vi "xdevice.vi"() -> ()   [LabVIEW 2019]
panel:
  out "GetDeviceInterface":refnum<k7>
  in  "stop":bool
  out "Device moved":bool
  in  "Wavelength":dbl=795.0
  out "Temperature":dbl
  out "Serial number":string
  out "Wavelength":dbl
  out "Angle":dbl
  out "Device detected":bool
  out "Error message":string
  in  "xphyspecLib.IXPhySpec":refnum<k7>
  # "Device status"
  # "Device information"
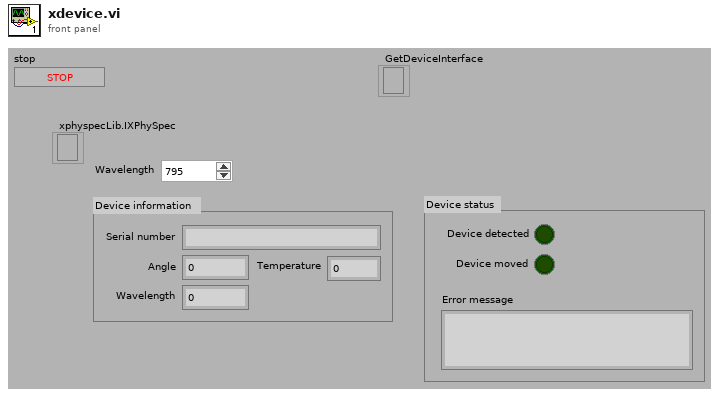
[diagram p1: front panel]
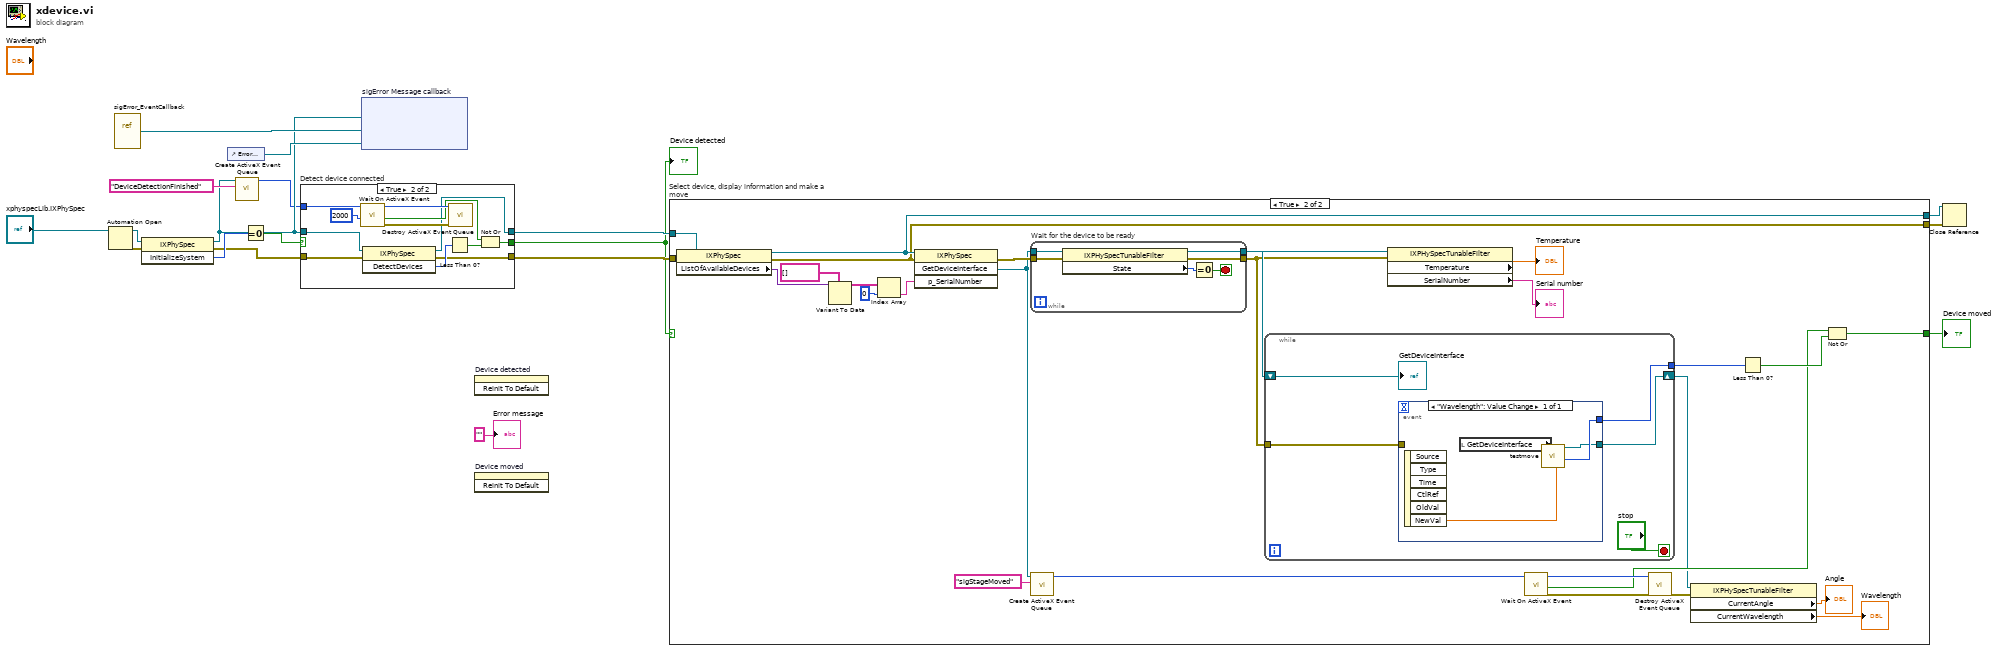
[diagram p0: block diagram]
diagram:
  n1 = Automation Open(Automation Refnum="xphyspecLib.IXPhySpec") -> (Automation Refnum=w17:refnum<k7>, error out=w16:errorcluster)  [unwired: 3 in]
  n2 = vi-ref "sigError_EventCallback.vi"() -> ("vi reference"=w13:refnum<vi>)
  n3 = invoke class="IXPhySpec" method="InitializeSystem"(reference=w17, error in=w16) -> (reference out=w10:refnum<k7>, error out=w9:errorcluster, "InitializeSystem"=w15:i32)  [unwired: 1 in]
  n4 = control-ref of="Error message"() -> (w14:refnum<vi>)
  n5 = call <vilib>:"Create ActiveX Event Queue.vi"("Event Name"="DeviceDetectionFinished", "Automation Refnum"=w10) -> ("Event Queue"=w8:i32)  [unwired: 4 in, 1 out]
  n6 = Equal To 0?(x=w15) -> (x = 0?=w11:bool)
  n7 = case "Detect device connected" shown="True" w11 {
    selector: w11 -> [w21 _]
    tunnel: w10 -> [w20 w33]
    tunnel: w9 -> [w19 w32]
    tunnel: w8 -> [_ w29]
    tunnel: [w20 w24] -> w7
    tunnel: [w19 w23] -> w6
    tunnel: [w21 w22] -> w5
    frame False {
    }
    frame True {
      n8 = call <vilib>:"Wait On ActiveX Event.vi"("ms Timeout (-1)"=2000, "Event Queue"=w29) -> ("error out"=w28:errorcluster, "Timed Out"=w26:bool, "Event Queue Out"=w30:i32)  [unwired: 2 in, 1 out]
      n9 = invoke class="IXPhySpec" method="DetectDevices"(reference=w33, error in=w32) -> (reference out=w24:refnum<k7>, error out=w23:errorcluster, "DetectDevices"=w27:i32)  [unwired: 1 in]
      n10 = Less Than 0?(x=w27) -> (x < 0?=w25:bool)
      n11 = call <vilib>:"Destroy ActiveX Event Queue.vi"("error in (no error)"=w28, "Event Queue"=w30) -> ()  [unwired: 5 in, 1 out]
      n12 = Not Or(1:w25, 2:w26) -> (0:w22:bool)
    }
  }
  "Device detected" <- w5
  n13 = node "sigError Message callback"(w10, w13, w14) -> ()  [unwired: 2 in, 2 out]
  n14 = invoke on="Device detected" class="Bool (strict)" method="Reinit To Default"() -> ()  [unwired: 3 in, 3 out]
  n15 = invoke on="Device moved" class="Bool (strict)" method="Reinit To Default"() -> ()  [unwired: 3 in, 3 out]
  n16 = case "Select device, display information and make a move" shown="True" w5 {
    selector: w5 -> [w36 _]
    tunnel: w7 -> [w35 w58]
    tunnel: w6 -> [w34 w57]
    tunnel: [w36 w45] -> w4
    tunnel: [w35 w44] -> w3
    tunnel: [w34 w43] -> w2
    frame False {
    }
    frame True {
      n17 = property class="IXPhySpec"(reference=w58, error in=w57) -> (reference out=w44:refnum<k7>, error out=w43:errorcluster, "ListOfAvailableDevices"=w60:variant)
      n18 = Variant To Data(type=string[] [], Variant=w60) -> (data=w62:string[])  [unwired: 1 in, 1 out]
      n19 = Index Array(array=w62, index=0) -> (element=w59:string)
      n20 = invoke class="IXPhySpec" method="GetDeviceInterface"(reference=w44, error in=w43, "p_SerialNumber"=w59) -> (error out=w56:errorcluster, "GetDeviceInterface"=w52:refnum<k7>)  [unwired: 1 in, 2 out]
      n21 = while "Wait for the device to be ready" {
        tunnel: [w76] -> w54
        tunnel: w52 -> [w74]
        tunnel: w56 -> [w75]
        tunnel: [w73] -> w55
        stop <- w77 stop-if-true
        n22 = property class="IXPHySpecTunableFilter"(reference=w74, error in=w75) -> (reference out=w73:refnum<k7>, error out=w76:errorcluster, "State"=w78:u32)
        n23 = Equal To 0?(x=w78) -> (x = 0?=w77:bool)
      }
      n24 = call <vilib>:"Create ActiveX Event Queue.vi"("Event Name"="sigStageMoved", "Automation Refnum"=w52) -> ("Event Queue"=w51:i32)  [unwired: 4 in, 1 out]
      n25 = while {
        tunnel: w54 -> [w68]
        tunnel: [w67] -> w48
        shift-right: [w66] -> w40
        shift-left: w55 -> [w64]
        stop <- "stop" stop-if-true
        n26 = event shown="[0] \"Wavelength\": Value Change" {
          selector: _ -> [_]
          dyn-events: _ -> [_]
          timeout: _ -> [_]
          tunnel: w68 -> [_]
          tunnel: [w70] -> w67
          tunnel: [w69] -> w66
          event "Wavelength": Value Change {
            n27 = event-data() -> ("NewVal"=w71:dbl)  [unwired: 1 in, 5 out]
            n28 = local read "GetDeviceInterface"() -> (w72:refnum<k7>)
            n29 = call "testmove.vi"("p_TargetWavelength"=w71, "reference"=w72) -> ("MovetoWavelength"=w70:i32, "reference out"=w69:refnum<k7>)  [unwired: 5 in, 3 out]
          }
        }
        "GetDeviceInterface" <- w64
      }
      n30 = property class="IXPHySpecTunableFilter"(reference=w55, error in=w54) -> ("Temperature"=→"Temperature":dbl, "SerialNumber"=→"Serial number":string)  [unwired: 2 out]
      n31 = call <vilib>:"Wait On ActiveX Event.vi"("Event Queue"=w51) -> ("error out"=w49:errorcluster, "Timed Out"=w46:bool, "Event Queue Out"=w50:i32)  [unwired: 3 in, 1 out]
      n32 = call <vilib>:"Destroy ActiveX Event Queue.vi"("error in (no error)"=w49, "Event Queue"=w50) -> ("error out"=w39:errorcluster)  [unwired: 5 in]
      n33 = property class="IXPHySpecTunableFilter"(reference=w40, error in=w39) -> ("CurrentAngle"=→"Angle":dbl, "CurrentWavelength"=→"Wavelength":dbl)  [unwired: 2 out]
      n34 = Less Than 0?(x=w48) -> (x < 0?=w47:bool)
      n35 = Not Or(1:w47, 2:w46) -> (0:w45:bool)
    }
  }
  "Device moved" <- w4
  n36 = Close Reference(reference=w3, error in (no error)=w2) -> ()  [unwired: 1 out]
  "Error message" <- "" ("Error message")
